vi "GetCryoInfo.vi"(11 "connection ID":refnum<k5>) -> (0 "User Stability":dbl, 1 "User Temp":dbl, 3 "connection ID out":refnum<k5>, 4 "Sample Stability":dbl, 6 "Sample Temp":dbl, 8 "Platform Stability":dbl, 9 "Platform Temp":dbl)   [LabVIEW 2019]
panel:
  out "Set Point":dbl
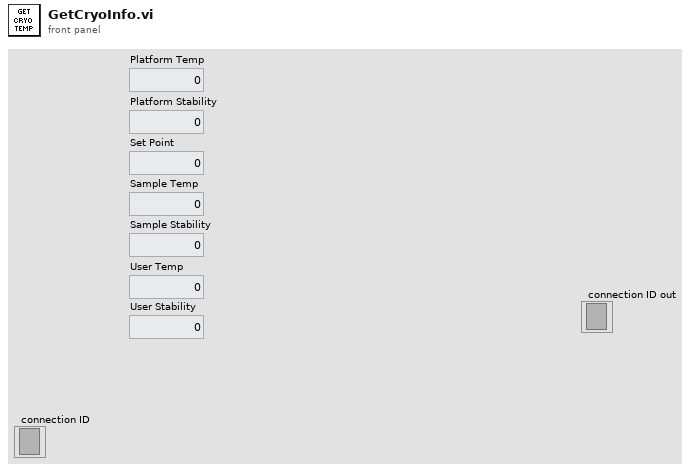
[diagram p1: front panel]
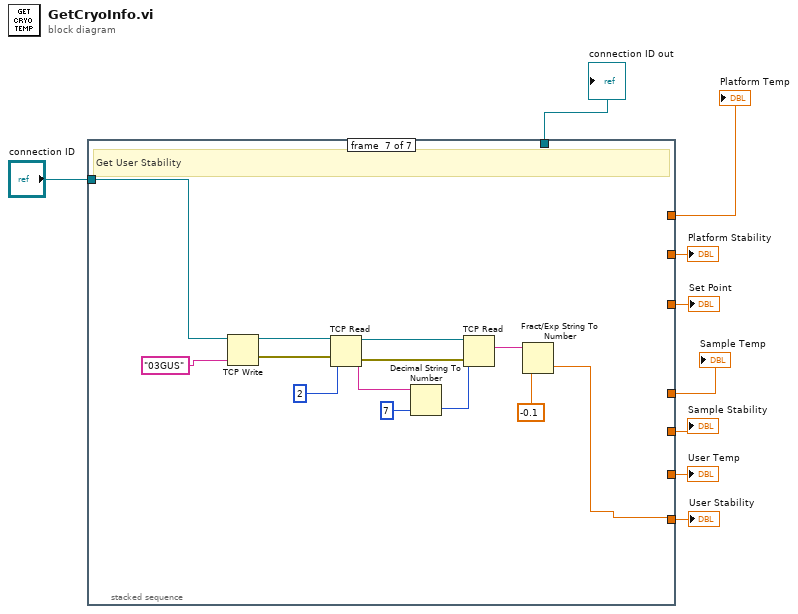
[diagram p0: block diagram]
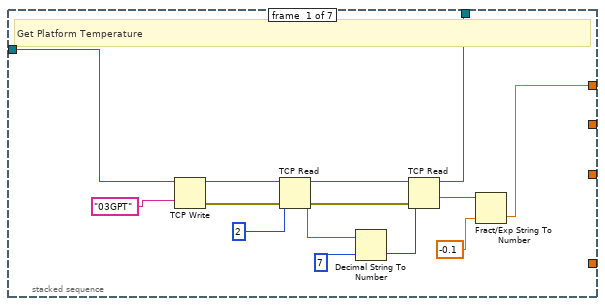
[diagram p2: hidden frame]
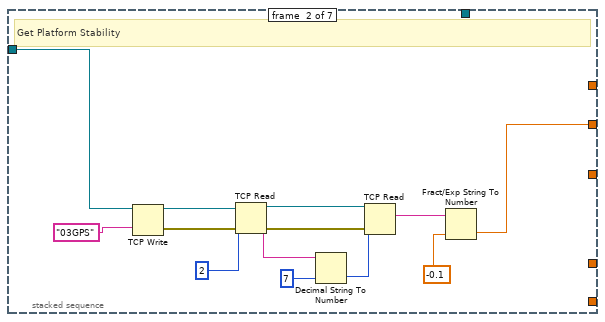
[diagram p3: hidden frame]
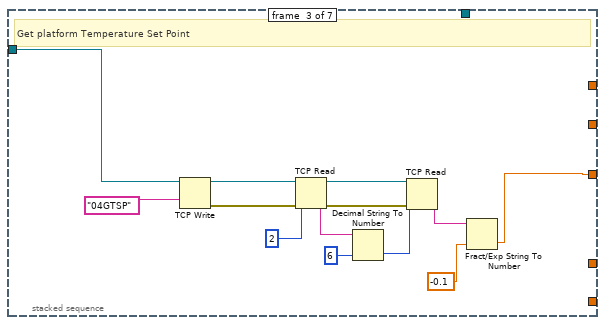
[diagram p4: hidden frame]
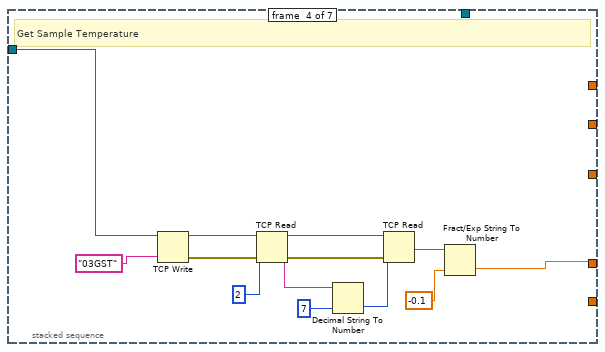
[diagram p5: hidden frame]
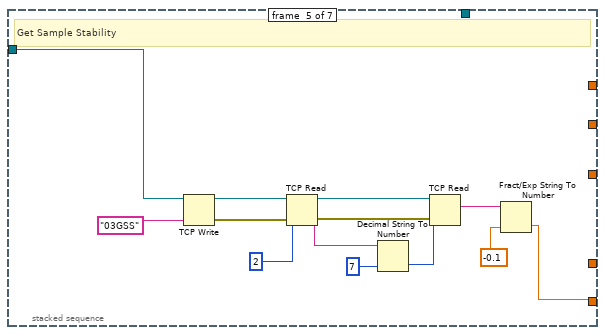
[diagram p6: hidden frame]
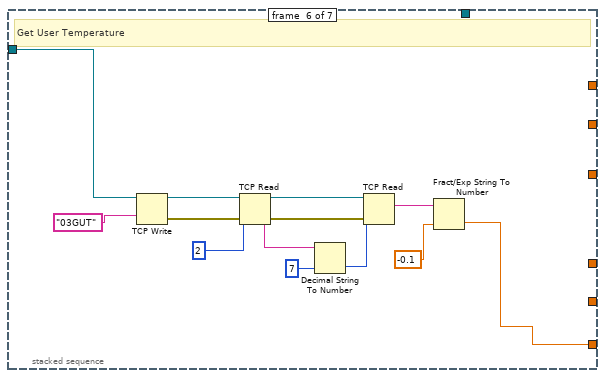
[diagram p7: hidden frame]
diagram:
  n1 = stacked-sequence {
    tunnel: "connection ID" -> [w20 w33 w46 w61 w72 w85 w98]
    tunnel: [_ _ w37 _ _ _ _] -> w5
    tunnel: [_ _ _ _ w63 _ _] -> w3
    tunnel: [w10 _ _ _ _ _ _] -> w7
    tunnel: [_ w24 _ _ _ _ _] -> w6
    tunnel: [_ _ _ w50 _ _ _] -> w4
    tunnel: [w15 _ _ _ _ _ _] -> w8
    tunnel: [_ _ _ _ _ w76 _] -> w2
    tunnel: [_ _ _ _ _ _ w89] -> w1
    frame #0 {
      # "Get Platform Temperature"
      n2 = TCP Write(connection ID=w20, data in="03GPT") -> (connection ID out=w23:refnum<k5>, error out=w14:errorcluster)  [unwired: 2 in, 1 out]
      n3 = TCP Read(connection ID=w23, bytes to read=2, error in (no error)=w14) -> (connection ID out=w18:refnum<k5>, data out=w19:string, error out=w13:errorcluster)  [unwired: 2 in]
      n4 = Decimal String To Number(string=w19, default (0L)=7 ("default (0 I32)")) -> (number=w17:i32)  [unwired: 1 in, 1 out]
      n5 = TCP Read(connection ID=w18, bytes to read=w17, error in (no error)=w13) -> (connection ID out=w15:refnum<k5>, data out=w16:string)  [unwired: 2 in, 1 out]
      n6 = Fract/Exp String To Number(string=w16, default (0 dbl)=-0.1 ("default (0 DBL)")) -> (number=w10:dbl)  [unwired: 2 in, 1 out]
    }
    frame #1 {
      # "Get Platform Stability"
      n7 = TCP Write(connection ID=w33, data in="03GPS") -> (connection ID out=w34:refnum<k5>, error out=w27:errorcluster)  [unwired: 2 in, 1 out]
      n8 = TCP Read(connection ID=w34, bytes to read=2, error in (no error)=w27) -> (connection ID out=w29:refnum<k5>, data out=w31:string, error out=w28:errorcluster)  [unwired: 2 in]
      n9 = Decimal String To Number(string=w31, default (0L)=7 ("default (0 I32)")) -> (number=w32:i32)  [unwired: 1 in, 1 out]
      n10 = TCP Read(connection ID=w29, bytes to read=w32, error in (no error)=w28) -> (data out=w30:string)  [unwired: 2 in, 2 out]
      n11 = Fract/Exp String To Number(string=w30, default (0 dbl)=-0.1 ("default (0 DBL)")) -> (number=w24:dbl)  [unwired: 2 in, 1 out]
    }
    frame #2 {
      # "Get platform Temperature Set Point"
      n12 = TCP Write(connection ID=w46, data in="04GTSP") -> (connection ID out=w47:refnum<k5>, error out=w41:errorcluster)  [unwired: 2 in, 1 out]
      n13 = TCP Read(connection ID=w47, bytes to read=2, error in (no error)=w41) -> (connection ID out=w44:refnum<k5>, data out=w45:string, error out=w40:errorcluster)  [unwired: 2 in]
      n14 = Decimal String To Number(string=w45, default (0L)=6 ("default (0 I32)")) -> (number=w43:i32)  [unwired: 1 in, 1 out]
      n15 = TCP Read(connection ID=w44, bytes to read=w43, error in (no error)=w40) -> (data out=w42:string)  [unwired: 2 in, 2 out]
      n16 = Fract/Exp String To Number(string=w42, default (0 dbl)=-0.1 ("default (0 DBL)")) -> (number=w37:dbl)  [unwired: 2 in, 1 out]
    }
    frame #3 {
      # "Get Sample Temperature"
      n17 = TCP Write(connection ID=w61, data in="03GST") -> (connection ID out=w59:refnum<k5>, error out=w54:errorcluster)  [unwired: 2 in, 1 out]
      n18 = TCP Read(connection ID=w59, bytes to read=2, error in (no error)=w54) -> (connection ID out=w57:refnum<k5>, data out=w58:string, error out=w53:errorcluster)  [unwired: 2 in]
      n19 = Decimal String To Number(string=w58, default (0L)=7 ("default (0 I32)")) -> (number=w56:i32)  [unwired: 1 in, 1 out]
      n20 = TCP Read(connection ID=w57, bytes to read=w56, error in (no error)=w53) -> (data out=w55:string)  [unwired: 2 in, 2 out]
      n21 = Fract/Exp String To Number(string=w55, default (0 dbl)=-0.1 ("default (0 DBL)")) -> (number=w50:dbl)  [unwired: 2 in, 1 out]
    }
    frame #4 {
      # "Get Sample Stability"
      n22 = TCP Write(connection ID=w72, data in="03GSS") -> (connection ID out=w75:refnum<k5>, error out=w67:errorcluster)  [unwired: 2 in, 1 out]
      n23 = TCP Read(connection ID=w75, bytes to read=2, error in (no error)=w67) -> (connection ID out=w70:refnum<k5>, data out=w71:string, error out=w66:errorcluster)  [unwired: 2 in]
      n24 = Decimal String To Number(string=w71, default (0L)=7 ("default (0 I32)")) -> (number=w69:i32)  [unwired: 1 in, 1 out]
      n25 = TCP Read(connection ID=w70, bytes to read=w69, error in (no error)=w66) -> (data out=w68:string)  [unwired: 2 in, 2 out]
      n26 = Fract/Exp String To Number(string=w68, default (0 dbl)=-0.1 ("default (0 DBL)")) -> (number=w63:dbl)  [unwired: 2 in, 1 out]
    }
    frame #5 {
      # "Get User Temperature"
      n27 = TCP Write(connection ID=w85, data in="03GUT") -> (connection ID out=w88:refnum<k5>, error out=w80:errorcluster)  [unwired: 2 in, 1 out]
      n28 = TCP Read(connection ID=w88, bytes to read=2, error in (no error)=w80) -> (connection ID out=w83:refnum<k5>, data out=w84:string, error out=w79:errorcluster)  [unwired: 2 in]
      n29 = Decimal String To Number(string=w84, default (0L)=7 ("default (0 I32)")) -> (number=w82:i32)  [unwired: 1 in, 1 out]
      n30 = TCP Read(connection ID=w83, bytes to read=w82, error in (no error)=w79) -> (data out=w81:string)  [unwired: 2 in, 2 out]
      n31 = Fract/Exp String To Number(string=w81, default (0 dbl)=-0.1 ("default (0 DBL)")) -> (number=w76:dbl)  [unwired: 2 in, 1 out]
    }
    frame #6 {
      # "Get User Stability"
      n32 = TCP Write(connection ID=w98, data in="03GUS") -> (connection ID out=w101:refnum<k5>, error out=w93:errorcluster)  [unwired: 2 in, 1 out]
      n33 = TCP Read(connection ID=w101, bytes to read=2, error in (no error)=w93) -> (connection ID out=w96:refnum<k5>, data out=w97:string, error out=w92:errorcluster)  [unwired: 2 in]
      n34 = Decimal String To Number(string=w97, default (0L)=7 ("default (0 I32)")) -> (number=w95:i32)  [unwired: 1 in, 1 out]
      n35 = TCP Read(connection ID=w96, bytes to read=w95, error in (no error)=w92) -> (data out=w94:string)  [unwired: 2 in, 2 out]
      n36 = Fract/Exp String To Number(string=w94, default (0 dbl)=-0.1 ("default (0 DBL)")) -> (number=w89:dbl)  [unwired: 2 in, 1 out]
    }
  }
  "connection ID out" <- w8
  "Platform Temp" <- w7
  "Platform Stability" <- w6
  "Set Point" <- w5
  "Sample Temp" <- w4
  "Sample Stability" <- w3
  "User Temp" <- w2
  "User Stability" <- w1
